vi "Log Data.vi"(7 "Command":T2=enum."Close", 8 "error in (no error)":errorcluster, 9 "Zone":i32, 10 "Status":T1, 11 "file path":path) -> (0 "error out":errorcluster)   [LabVIEW 2013]
doc: "This subVI is use to log the data to the Security log.txt file\nIt is -\n-Initializing the file path\n-Write the data\n-Stop the file path."
uses:
  Controls/Security log States.ctl
  Controls/Security Zones.ctl
  <vilib>/Utility/file.llb/Write To Spreadsheet File (string).vi
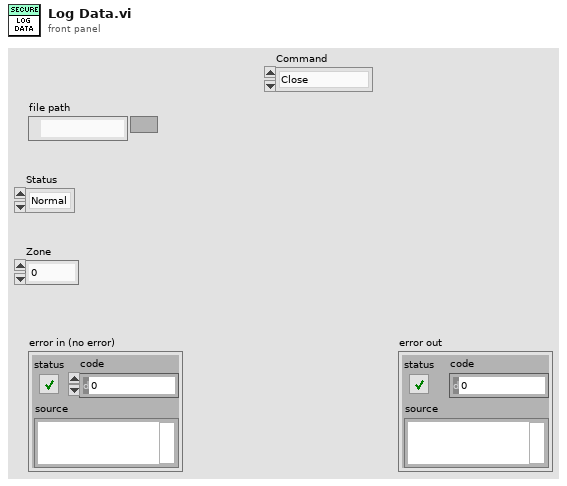
[diagram p1: front panel]
types:
  T1 = typedef "Security Zones.ctl" = enum16{"Normal", "Alarm", "Bypass", "Tamper"}
  T2 = typedef "Security log States.ctl" = enum16{"Initialize", "Write", "Close"}
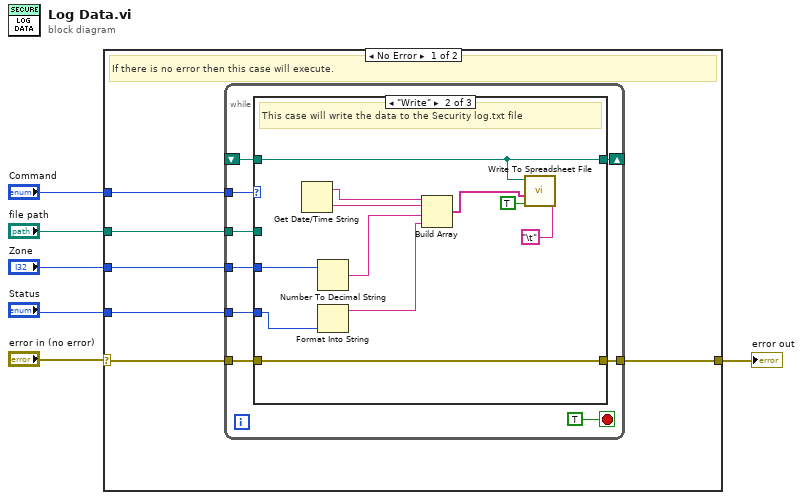
[diagram p0: block diagram]
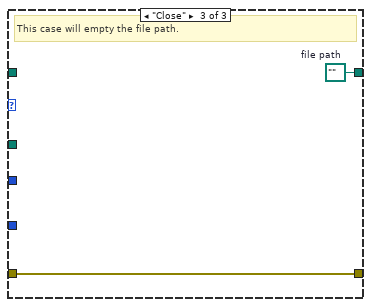
[diagram p3: hidden frame]
diagram:
  n1 = case shown="No Error" "error in (no error)" {
    selector: "error in (no error)" -> [w9 w37]
    tunnel: "Command" -> [w12 _]
    tunnel: "file path" -> [w7 _]
    tunnel: "Status" -> [w11 _]
    tunnel: "Zone" -> [w10 _]
    tunnel: [w8 w37] -> w6
    frame No Error {
      # "If there is no error then this case will execute."
      n2 = while {
        tunnel: w12 -> [w20]
        tunnel: w7 -> [w19]
        shift-right: [w18] -> _
        shift-left: _ -> [w17]
        tunnel: w11 -> [w16]
        tunnel: w10 -> [w15]
        tunnel: w9 -> [w14]
        tunnel: [w13] -> w8
        stop <- TRUE stop-if-true
        n3 = case shown="\"Write\"" w20 {
          tunnel: w19 -> [w23 _ _]
          tunnel: [w23 w34 w36] -> w18
          tunnel: w17 -> [_ w34 _]
          tunnel: w16 -> [_ w25 _]
          tunnel: w15 -> [_ w31 _]
          tunnel: w14 -> [w22 w30 w35]
          tunnel: [w22 w30 w35] -> w13
          frame "Initialize", Default {
            # "Stoaring the file path to the shift register."
            # "This case will initialize the file path."
          }
          frame "Write" {
            # "This case will write the data to the Security log.txt file"
            n4 = Get Date/Time String() -> (date string=w33:string, time string=w32:string)  [unwired: 3 in]
            n5 = Number To Decimal String(number=w31) -> (decimal integer string=w26:string)  [unwired: 1 in]
            n6 = Format Into String(w25) -> (resulting string=w24:string)  [unwired: 3 in, 1 out]
            n7 = Build Array(w33, w32, w26, w24) -> (w27:string[])
            n8 = call-poly <vilib>:"Write To Spreadsheet File.vi"("delimiter (\\t)"="\t", "append to file? (new file:F)"=TRUE, "1D data"=w27, "file path (dialog if empty)"=w34) -> ()  [unwired: 4 in, 1 out]
          }
          frame "Close" {
            w36 = path ""  # file path
            # "This case will empty the file path."
          }
        }
      }
    }
    frame Error {
      # "If there is error then this case will execute."
    }
  }
  "error out" <- w6
